vi "waveform_conversion.vi"(10 "sample length":i32, 11 "Array":waveform(dbl)[](array[waveform])) -> (3 "mean":dbl)   [LabVIEW 2026]
uses:
  <vilib>/ptbypt/NI_PtbyPt.lvlib
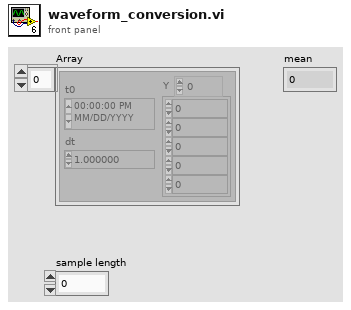
[diagram p1: front panel]
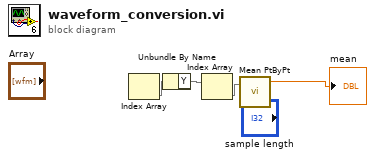
[diagram p0: block diagram]
diagram:
  n1 = Index Array() -> (element=w1)  [unwired: 2 in]
  n2 = Unbundle By Name(w1) -> ("Y"=w3)
  n3 = Index Array(array=w3) -> (element=w4)  [unwired: 1 in]
  n4 = call <vilib>:"Mean PtByPt.vi"("x"=w4, "sample length"="sample length") -> ("mean"=→"mean":dbl)  [unwired: 2 in, 1 out]
